vi "example_08_confirmation_input.vi"() -> ()   [LabVIEW 2015, in "lv-dialog.lvlib" / "v1.lvlib"]
uses:
  v1.lvlib
  public/class/v1.lvclass
  public/_controls/selection.ctl
panel:
  in  "boolean_text_2":string="Cancel"
  in  "boolean_text_1":string="DELETE"
  in  "dialog_text":string="DELETE"
  out "error out":errorcluster
  out "dialog_selection":T1
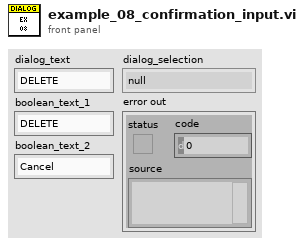
[diagram p1: front panel]
types:
  T1 = typedef "lv-dialog.lvlib/v1.lvlib/selection.ctl" = enum16{"null", "panel_closed", "button_1", "button_2", "button_3", "cancelled"}
  T2 = cluster{"dialog_text":string, "boolean_text_1":string, "boolean_text_2":string}
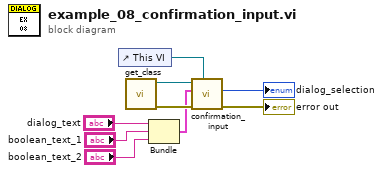
[diagram p0: block diagram]
diagram:
  n1 = control-ref of="This VI"() -> (w9:refnum<vi>)
  n2 = call "get_class.vi"() -> ("error out"=w5:errorcluster, "class"=w6:refnum<class "v1.lvclass">)  [unwired: 10 in]
  n3 = Bundle("dialog_text"="dialog_text", "boolean_text_1"="boolean_text_1", "boolean_text_2"="boolean_text_2") -> (w4:T2)  [unwired: 1 in]
  n4 = call-dynamic "confirmation_input.vi"("callee"=w9, "error in (no error)"=w5, "configuration"=w4, "v1 in"=w6) -> ("error out"=→"error out":errorcluster, "dialog_selection"=→"dialog_selection":T1)  [unwired: 5 in, 1 out]
